vi "Read motor pos notifier.vi"(11 "Motor in":refnum<class "Motor.lvclass">) -> (2 "motor pos notifier":refnum<notifier>, 3 "Motor out":refnum<class "Motor.lvclass">)   [LabVIEW 2016, in "Hardware.lvlib" / "Motor.lvlib" / "Motor.lvclass"]
uses:
  <userlib>/Common Components/Hardware/Motor/Motor/Motor.lvclass
  <userlib>/Common Components/Hardware/Motor/Motor/Motor.lvclass/Motor.ctl
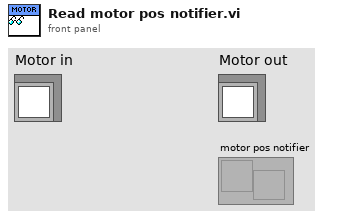
[diagram p1: front panel]
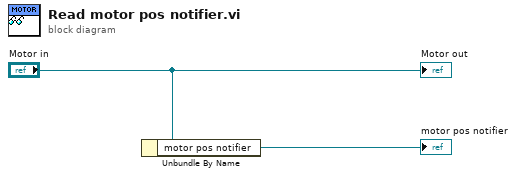
[diagram p0: block diagram]
diagram:
  n1 = Unbundle By Name("Motor in") -> ("motor pos notifier"=→"motor pos notifier":refnum<notifier>)
  "Motor out" <- "Motor in"
